vi "Initialize Drive.vi"   [LabVIEW 2017]
uses:
  Globals/Robot Global Data.vi
  <vilib>/Rock Robotics/WPI/RobotDrive/WPI_RobotDriveOpen2MotorWithExistingMotors.vi
types:
  T1 = typedef "WPI_MotorControlDeviceRef.ctl" = cluster{"DeviceStatus":errorcluster, "Type":T2, "PWM":cluster{"PWM Channel":T3, "DeadBand":T4}, "CAN":cluster{"Device Number":u8, "SetOutput VI Ref":variant, "GetOutput VI Ref":variant, "Enable VI Ref":variant, "Disable VI Ref":variant, "Data":variant}, "Invert":bool, "DIO PWM":cluster{"PWM \"Enable\" Channel":T3, "DIOChannel":T5, "PWM Rate":dbl}}
  T2 = typedef "WPI_MotorControlType.ctl" = enum16{"PWM", "CAN", "DIO PWM"}
  T3 = typedef "FPGA_DIOPWMChannel.ctl" = enum8{"PWM 0", "PWM 1", "PWM 2", "PWM 3", "PWM 4", "PWM 5", "PWM 6", "PWM 7", "PWM 8", "PWM 9", "PWM MXP 0", "PWM MXP 1", "PWM MXP 2", "PWM MXP 3", "PWM MXP 4", "PWM MXP 5", "PWM MXP 6", "PWM MXP 7", "PWM MXP 8", "PWM MXP 9", "Invalid"}
  T4 = typedef "WPI_PWMDeadband.ctl" = cluster{"Name":string, "maxPositivePwm":i32, "minPositivePwm":i32, "centerPwm":i32, "maxNegativePwm":i32, "minNegativePwm":i32, "angularRange":u16}
  T5 = typedef "FPGA_DIOChannel.ctl" = enum8{"DIO 0", "DIO 1", "DIO 2", "DIO 3", "DIO 4", "DIO 5", "DIO 6", "DIO 7", "DIO 8", "DIO 9", "DIO MXP 0", "DIO MXP 1", "DIO MXP 2", "DIO MXP 3", "DIO MXP 4", "DIO MXP 5", "DIO MXP 6", "DIO MXP 7", "DIO MXP 8", "DIO MXP 9", "DIO MXP 10", "DIO MXP 11", "DIO MXP 12", "DIO MXP 13", "DIO MXP 14", "DIO MXP 15", "SPI Port CS1", "SPI Port CS2", "SPI Port CS3", "SPI Port MISO", "SPI Port MOSI", "Invalid"}
  T6 = typedef "WPI_RobotDriveDevRef.ctl" = cluster{"DevStatus":errorcluster, "Motors[]":T1[], "Square Inputs":bool, "Max Output":dbl}
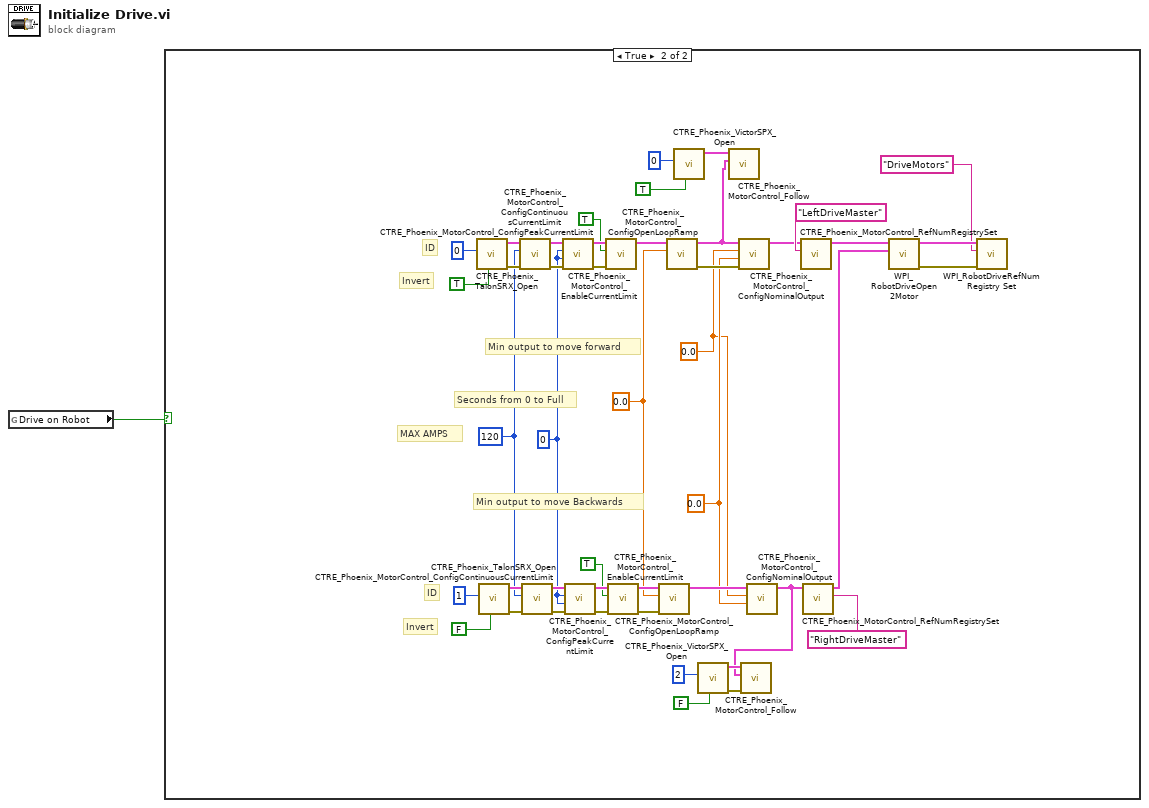
[diagram p0: block diagram]
diagram:
  n1 = global read "Robot Global Data.vi" "Drive on Robot"() -> (w1:bool)
  n2 = case shown="True" w1 {
    frame False {
    }
    frame True {
      w11 = 0.0 ("Forward Nominal Percent Output")
      w12 = 0.0 ("Reverse Nominal Percent Output")
      w16 = 0.0 ("secondsFromNeutralToFull")
      w24 = 0 ("Peak Current (Amps)")
      w25 = 120 ("Continuous Current Limit (Amps)")
      # "Min output to move Backwards"
      # "Min output to move forward"
      # "Seconds from 0 to Full"
      # "ID"
      # "ID"
      # "Invert"
      # "Invert"
      # "MAX AMPS"
      n3 = call "CTRE_Phoenix_TalonSRX_Open.vi"("Invert"=TRUE, "Device Number"=u8 0) -> ("error out"=w45:errorcluster, "CAN Talon SRX Ref"=w44:T1)  [unwired: 8 in]
      n4 = call "CTRE_Phoenix_TalonSRX_Open.vi"("Invert"=FALSE, "Device Number"=u8 1) -> ("error out"=w32:errorcluster, "CAN Talon SRX Ref"=w33:T1)  [unwired: 8 in]
      n5 = call "CTRE_Phoenix_MotorControl_ConfigContinuousCurrentLimit.vi"("error in (no error)"=w45, "Continuous Current Limit (Amps)"=w25, "PhoenixMotorControlDevRef"=w44) -> ("error out"=w43:errorcluster, "PhoenixMotorControlDevRef"=w42:T1)  [unwired: 7 in]
      n6 = call "CTRE_Phoenix_MotorControl_ConfigContinuousCurrentLimit.vi"("error in (no error)"=w32, "Continuous Current Limit (Amps)"=w25, "PhoenixMotorControlDevRef"=w33) -> ("error out"=w34:errorcluster, "PhoenixMotorControlDevRef"=w35:T1)  [unwired: 7 in]
      n7 = call "CTRE_Phoenix_MotorControl_ConfigPeakCurrentLimit.vi"("error in (no error)"=w43, "Peak Current Maximum Duration (ms)"=w24, "Peak Current (Amps)"=w24, "PhoenixMotorControlDevRef"=w42) -> ("error out"=w41:errorcluster, "PhoenixMotorControlDevRef"=w40:T1)  [unwired: 6 in]
      n8 = call "CTRE_Phoenix_MotorControl_ConfigPeakCurrentLimit.vi"("error in (no error)"=w34, "Peak Current Maximum Duration (ms)"=w24, "Peak Current (Amps)"=w24, "PhoenixMotorControlDevRef"=w35) -> ("error out"=w36:errorcluster, "PhoenixMotorControlDevRef"=w37:T1)  [unwired: 6 in]
      n9 = call "CTRE_Phoenix_MotorControl_EnableCurrentLimit.vi"("error in (no error)"=w41, "Enable Current Limit?"=TRUE, "PhoenixMotorControlDevRef"=w40) -> ("PhoenixMotorControlDevRef"=w17:T1)  [unwired: 7 in, 1 out]
      n10 = call "CTRE_Phoenix_MotorControl_EnableCurrentLimit.vi"("error in (no error)"=w36, "Enable Current Limit?"=TRUE, "PhoenixMotorControlDevRef"=w37) -> ("error out"=w19:errorcluster, "PhoenixMotorControlDevRef"=w18:T1)  [unwired: 7 in]
      n11 = call "CTRE_Phoenix_MotorControl_ConfigOpenLoopRamp.vi"("error in (no error)"=w19, "secondsFromNeutralToFull"=w16, "PhoenixMotorControlDevRef"=w18) -> ("PhoenixMotorControlDevRef"=w14:T1)  [unwired: 7 in, 1 out]
      n12 = call "CTRE_Phoenix_MotorControl_ConfigOpenLoopRamp.vi"("secondsFromNeutralToFull"=w16, "PhoenixMotorControlDevRef"=w17) -> ("error out"=w15:errorcluster, "PhoenixMotorControlDevRef"=w2:T1)  [unwired: 8 in]
      n13 = call "CTRE_Phoenix_VictorSPX_Open.vi"("Invert"=TRUE, "Device Number"=u8 0) -> ("CAN Talon SRX Ref"=w9:T1)  [unwired: 8 in, 1 out]
      n14 = call "CTRE_Phoenix_VictorSPX_Open.vi"("Invert"=FALSE, "Device Number"=u8 2) -> ("error out"=w5:errorcluster, "CAN Talon SRX Ref"=w6:T1)  [unwired: 8 in]
      n15 = call "CTRE_Phoenix_MotorControl_Follow.vi"("Master Controller to Follow"=w2, "PhoenixMotorControlDevRef"=w9) -> ()  [unwired: 8 in, 2 out]
      n16 = call "CTRE_Phoenix_MotorControl_ConfigNominalOutput.vi"("error in (no error)"=w15, "Reverse Nominal Percent Output"=w12, "Forward Nominal Percent Output"=w11, "PhoenixMotorControlDevRef"=w2) -> ("PhoenixMotorControlDevRef"=w13:T1)  [unwired: 6 in, 1 out]
      n17 = call "CTRE_Phoenix_MotorControl_ConfigNominalOutput.vi"("Reverse Nominal Percent Output"=w12, "Forward Nominal Percent Output"=w11, "PhoenixMotorControlDevRef"=w14) -> ("PhoenixMotorControlDevRef"=w3:T1)  [unwired: 7 in, 1 out]
      n18 = call "CTRE_Phoenix_MotorControl_Follow.vi"("error in (no error)"=w5, "Master Controller to Follow"=w3, "PhoenixMotorControlDevRef"=w6) -> ()  [unwired: 7 in, 2 out]
      n19 = call <vilib>:"CTRE_Phoenix_MotorControl_RefNumRegistrySet.vi"("refnum name"="LeftDriveMaster", "PhoenixMotorControlDevRef"=w13) -> ("PhoenixMotorControlDevRef"=w30:T1)  [unwired: 8 in, 1 out]
      n20 = call <vilib>:"CTRE_Phoenix_MotorControl_RefNumRegistrySet.vi"("refnum name"="RightDriveMaster", "PhoenixMotorControlDevRef"=w3) -> ("PhoenixMotorControlDevRef"=w29:T1)  [unwired: 8 in, 1 out]
      n21 = call-poly <vilib>:"WPI_RobotDriveOpen2Motor.vi"("Right Motor Dev Ref"=w29, "Left Motor Dev Ref"=w30) -> ("error out"=w28:errorcluster, "RobotDriveDevRef"=w27:T6)  [unwired: 8 in]
      n22 = call <vilib>:"WPI_RobotDriveRefNum Registry Set.vi"("error in (no error)"=w28, "refnum name"="DriveMotors", "RobotDriveDevRef"=w27) -> ()  [unwired: 7 in, 2 out]
    }
  }
